vi "Read Default From File.vi"(8 "error in (no error)":errorcluster, 9 "Name":string, 10 "Path":path, 11 "Rectangle Settings in":refnum<class "Rectangle Settings.lvclass">) -> (0 "error out":errorcluster, 3 "Rectangle Settings out":refnum<class "Rectangle Settings.lvclass">)   [LabVIEW 2019, in "Rectangle Settings.lvclass"]
uses:
  Rectangle Settings.lvclass
  ObjectSettings/ObjectSettings.lvclass
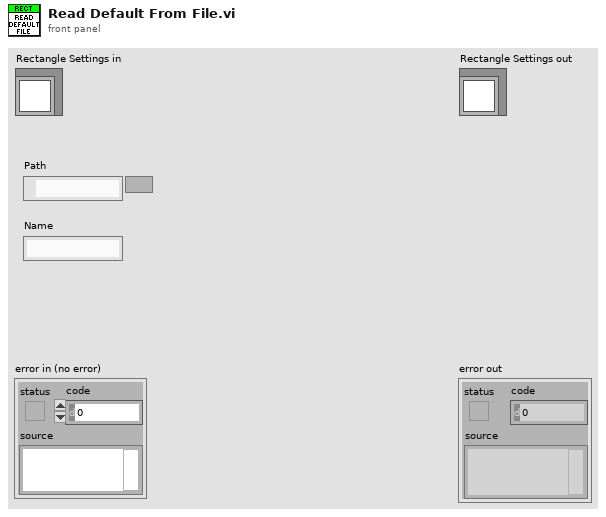
[diagram p1: front panel]
types:
  T1 = typedef "Rectangle Settings.lvclass/Default Rectangle Cluster.ctl" = cluster{"Fill Orientation":u16, "Fill Spacing":dbl}
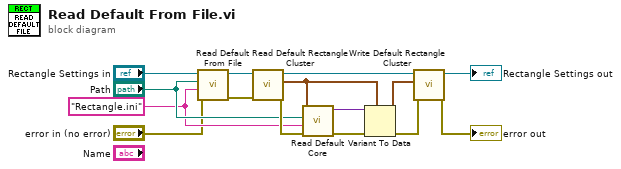
[diagram p0: block diagram]
diagram:
  w3 = "Rectangle.ini"
  n1 = call-parent "Read Default From File.vi"("error in (no error)"="error in (no error)", "Name"=w3, "Path"="Path", "ObjectSettings in"="Rectangle Settings in") -> ("error out"=w9:errorcluster, "ObjectSettings out"=w11:refnum<class "Rectangle Settings.lvclass">)  [unwired: 6 in]
  n2 = call "Read Default Rectangle Cluster.vi"("error in (no error)"=w9, "Rectangle Settings in"=w11) -> ("error out"=w7:errorcluster, "Default Rectangle Cluster"=w5:T1, "Rectangle Settings out"=w10:refnum<class "Rectangle Settings.lvclass">)  [unwired: 7 in]
  n3 = call "Read Default Core.vi"("error in (no error)"=w7, "Name"=w3, "Path"="Path", "Cluster In"=w5) -> ("error out"=w14:errorcluster, "Cluster Out"=w6:variant)  [unwired: 6 in]
  n4 = Variant To Data(error in=w14, type=w5, Variant=w6) -> (data=w12:T1, error out=w8:errorcluster)
  n5 = call "Write Default Rectangle Cluster.vi"("error in (no error)"=w8, "Default Rectangle"=w12, "Rectangle Settings in"=w10) -> ("error out"=→"error out":errorcluster, "Rectangle Settings out"=→"Rectangle Settings out":refnum<class "Rectangle Settings.lvclass">)  [unwired: 7 in]
